vi "main.vi"() -> ()   [LabVIEW 2020]
uses:
  FGVs/FGVstates.ctl
panel:
  in  "error in (no error)":errorcluster
  out "error out":errorcluster
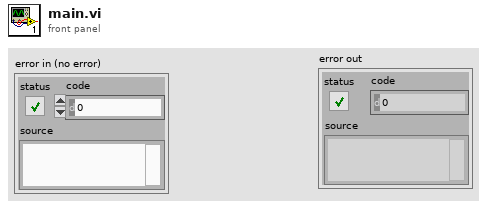
[diagram p1: front panel]
types:
  T1 = typedef "FGVstates.ctl" = enum16{"Init", "Set", "Get", "De-Init"}
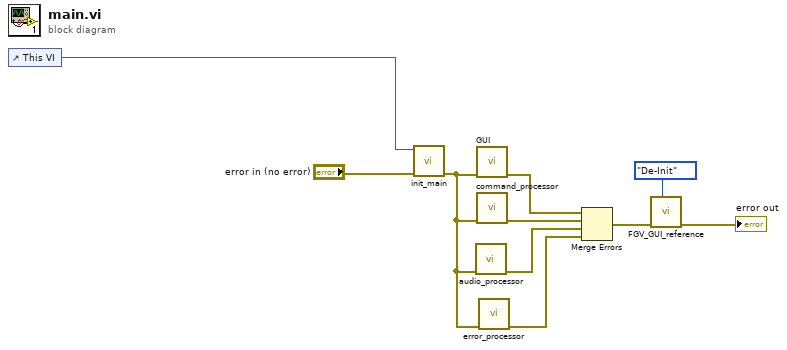
[diagram p0: block diagram]
diagram:
  n1 = control-ref of="This VI"() -> (w6:refnum<vi>)
  n2 = call "init_main.vi"("error in (no error)"="error in (no error)", "VI in"=w6) -> ("error out"=w4:errorcluster)  [unwired: 9 in]
  n3 = call "audio_processor.vi"("error in (no error)"=w4) -> ("error out"=w8:errorcluster)  [unwired: 10 in]
  n4 = call "GUI.vi"("error in (no error)"=w4) -> ("error out"=w10:errorcluster)  [unwired: 10 in]
  n5 = call "command_processor.vi"("error in (no error)"=w4) -> ("error out"=w9:errorcluster)  [unwired: 10 in]
  n6 = call "error_processor.vi"("error in (no error)"=w4) -> ("error out"=w7:errorcluster)  [unwired: 10 in]
  n7 = Merge Errors(w10, w9, w8, w7) -> (w2:errorcluster)
  n8 = call "FGV_GUI_reference.vi"("FGV states"=FGVstates."De-Init", "error in (no error)"=w2) -> ("error out"=→"error out":errorcluster)  [unwired: 8 in, 1 out]
